vi "novoGoleiroAlinharComATrave.vi"(8 "balls":T1[](array[typedef]), 9 "Robot in":T2, 10 "Goleiro.X_padrao":dbl, 11 "IA State":T7={"our_robots"=[], "enemy_robots"=[], "balls"=[], "geometry"={"field_length"=0, "field_width"=0, "goal_width"=0, "goal_depth"=0, "center_circle_radius"=0, "defense_width"=0, "defense_depth"=0, "free_kick_from_defense_dist"=0, "penalty_spot_from_field_line_dist"=0, "penalty_line_from_spot_dist"=0, "half_moon_depth"=0, "half_moon_width"=0}, "IA Judge"={"stage"="", "command"="", "our_goalie_id"=0.0, "enemy_goalie_id"=0.0, "command enum"=enum."Halt", "Time"=enum."Azul"}, "Received Timestamp"=timestamp(0 s since 1904-01-01), "Events"={"Touch"=FALSE, "id touch"=0.0, "Ball out of \nVision"=FALSE, "Ball inside \nGoalie area"=FALSE, "Robot not responding"=FALSE, "Robots responding status"=[1.0, 1.0, 1.0, 1.0, 1.0, 1.0], "Enemy Ball \nPossession"=FALSE, "Id ini Possession"=0.0, "Ball Possesion"=FALSE, "Id Possesion"=0.0, "Ball at\nour goal side"=FALSE, "Ball at\ntouchline"=FALSE, "Ball at\nenemy goal side"=FALSE}}) -> (3 "Cluster de saída":T2)   [LabVIEW 2018]
uses:
  Core/AI Input.ctl
  Core/AI Robot.ctl
  Intel/Functions Enum.ctl
  Intel/AttackerStates.ctl
  Path Planning/RRT/PathDests.ctl
  Path Planning/RRT/PathDest.ctl
  Core/AI Ball.ctl
  Core/Field Size.ctl
  Core/AI Judge.ctl
  Intel/Command Enum.ctl
  Util/Events/Events.ctl
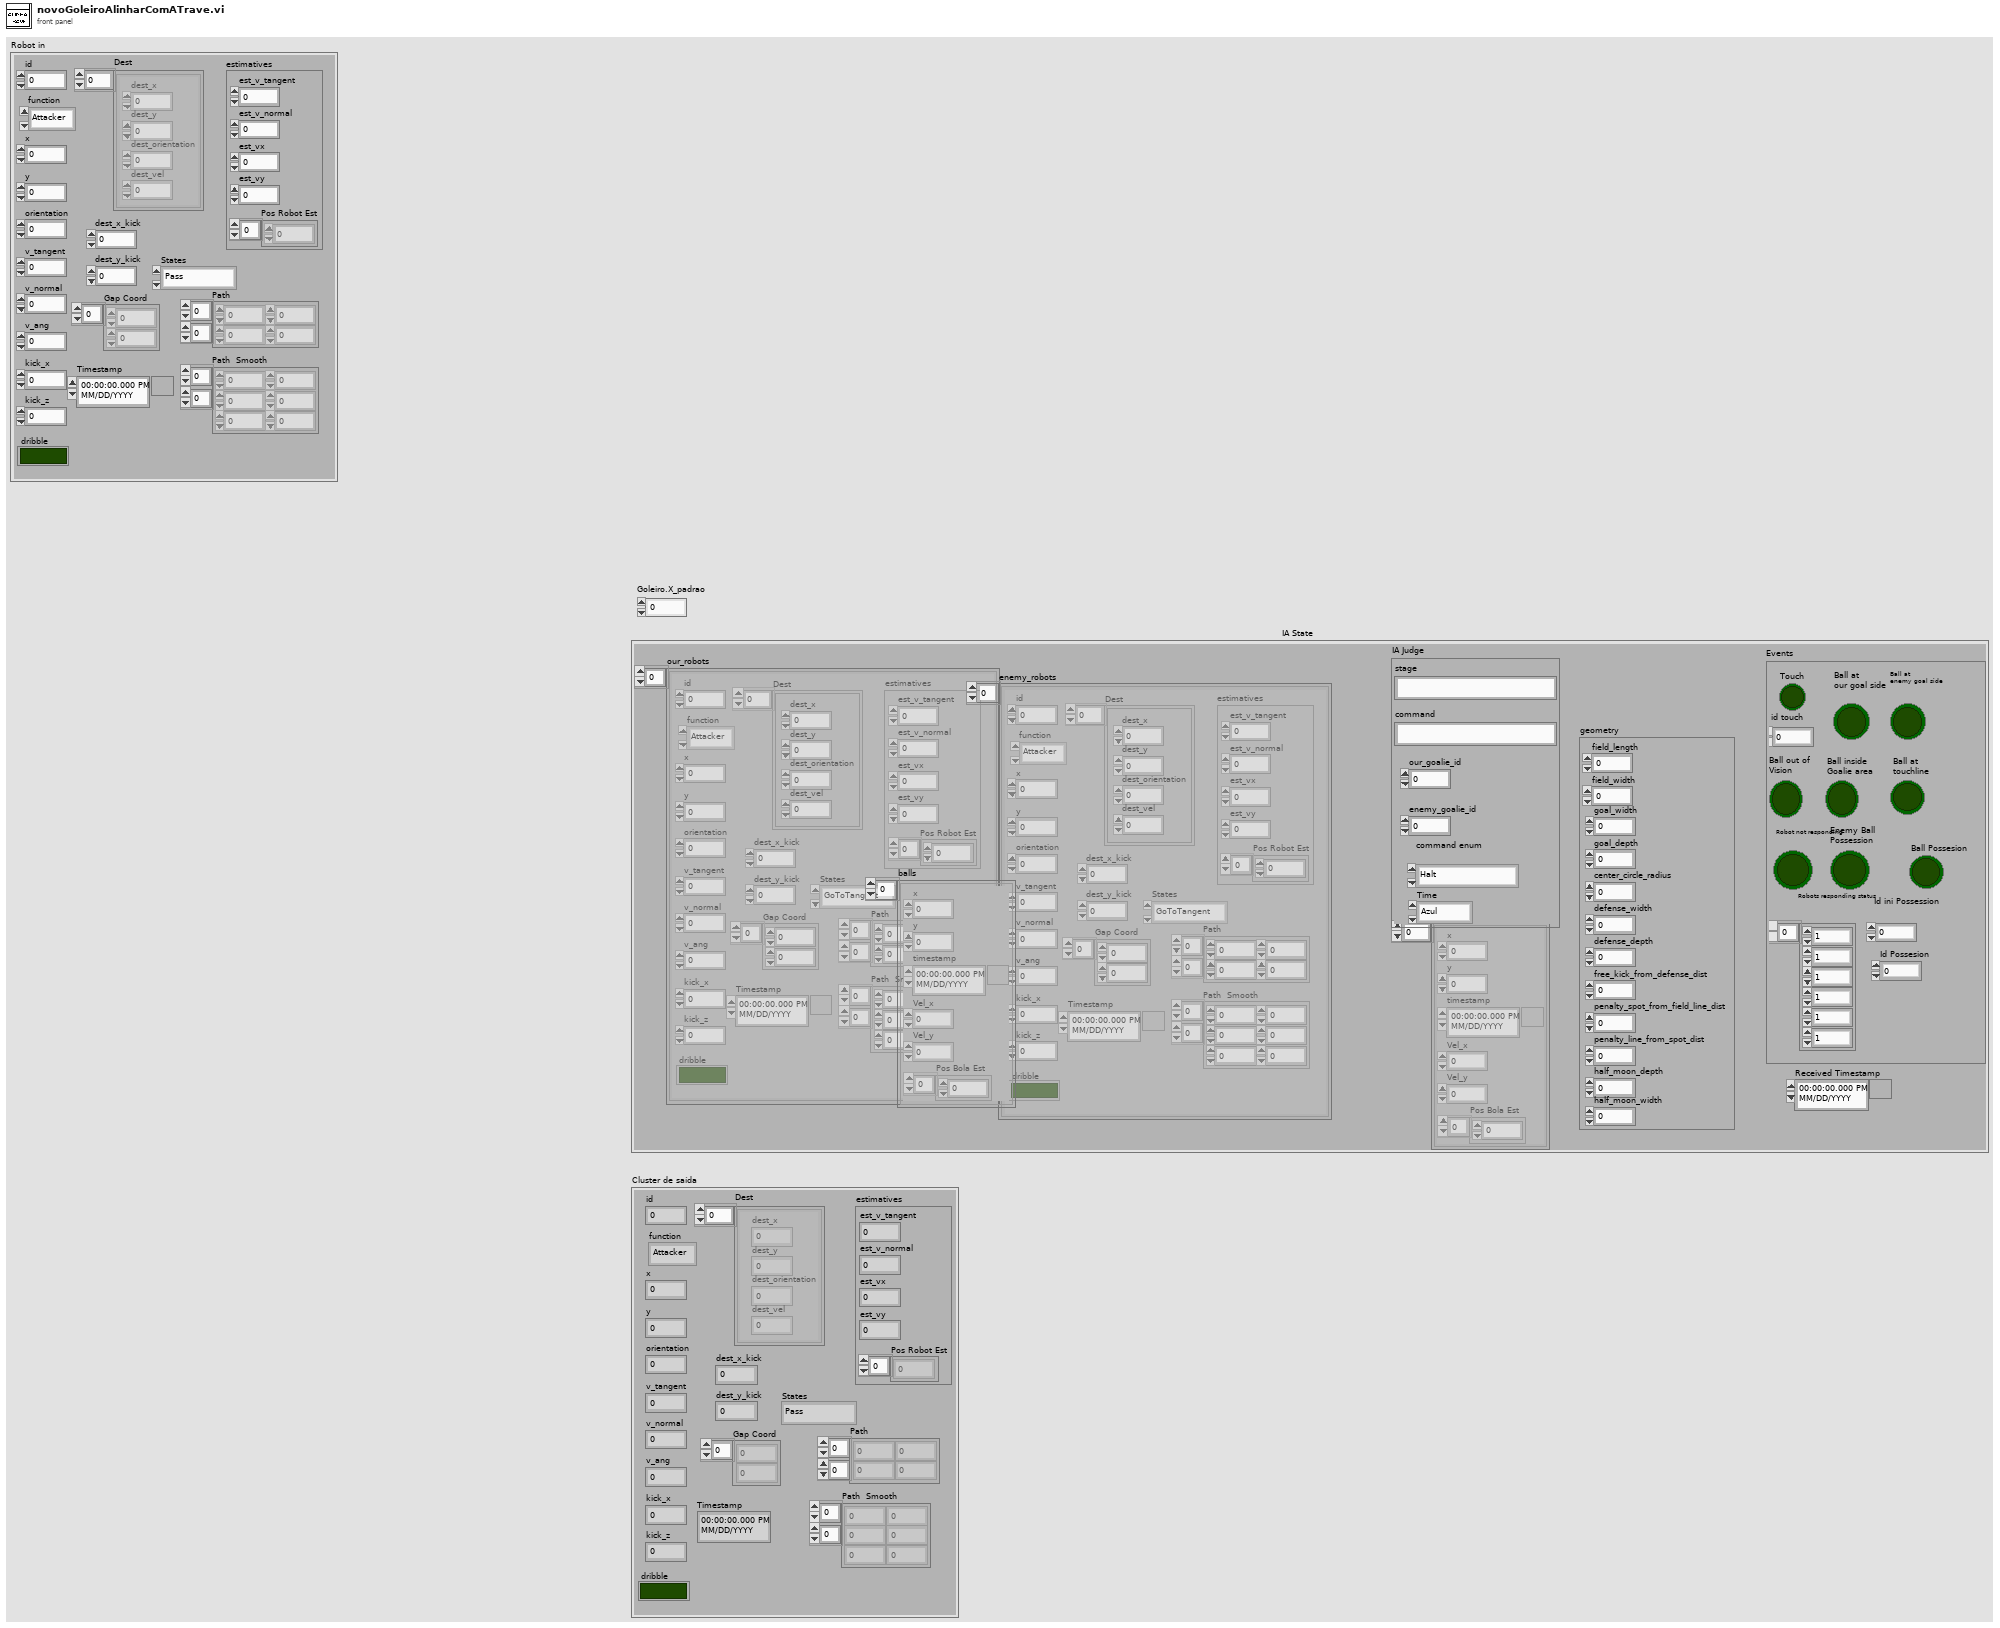
[diagram p1: front panel]
types:
  T1 = typedef "AI Ball.ctl" = cluster{"x":dbl, "y":dbl, "timestamp":timestamp, "Vel_x":dbl, "Vel_y":dbl, "Pos Bola Est":dbl[]}
  T2 = typedef "AI Robot.ctl" = cluster{"id":u32, "function":T3, "x":dbl, "y":dbl, "orientation":dbl, "v_tangent":dbl, "v_normal":dbl, "v_ang":dbl, "kick_x":dbl, "kick_z":dbl, "dribble":bool, "Timestamp":timestamp, "estimatives":cluster{"est_v_tangent":dbl, "est_v_normal":dbl, "est_vx":dbl, "est_vy":dbl, "Pos Robot Est":dbl[]}, "dest_x_kick":dbl, "dest_y_kick":dbl, "Gap Coord":dbl[], "States":T4, "Path ":dbl[][], "Path  Smooth":dbl[][], "Dest":T5}
  T3 = typedef "Functions Enum.ctl" = enum16{"Attacker", "Goalie", "Defender", "Striker", "Goto 0", "Dummy", "Kicker", "ZigZag"}
  T4 = typedef "AttackerStates.ctl" = enum16{"Pass", "GoToTangent", "BallGetting", "GoToKick", "Rotate anti-clockwise", "Rotate Clockwise", ""}
  T5 = typedef "PathDests.ctl" = T6[]
  T6 = typedef "PathDest.ctl" = cluster{"dest_x":dbl, "dest_y":dbl, "dest_orientation":dbl, "dest_vel":dbl}
  T7 = typedef "AI Input.ctl" = cluster{"our_robots":T2[], "enemy_robots":T2[], "balls":T1[], "geometry":T8, "IA Judge":T9, "Received Timestamp":timestamp, "Events":T11}
  T8 = typedef "Field Size.ctl" = cluster{"field_length":u32, "field_width":u32, "goal_width":u32, "goal_depth":u32, "center_circle_radius":u32, "defense_width":u32, "defense_depth":u32, "free_kick_from_defense_dist":u32, "penalty_spot_from_field_line_dist":u32, "penalty_line_from_spot_dist":u32, "half_moon_depth":u32, "half_moon_width":u32}
  T9 = typedef "AI Judge.ctl" = cluster{"stage":string, "command":string, "our_goalie_id":dbl, "enemy_goalie_id":dbl, "command enum":T10, "Time":enum16{"Azul", "Amarelo"}}
  T10 = typedef "Command Enum.ctl" = enum16{"Halt", "Stop", "Force Start", "PKA Normal Start", "Prepare Kickoff Ally", "PKE Normal Start", "Prepare Kickoff Enemy", "Prepare Penalty Ally", "PPA Normal Start", "Prepare Penalty Enemy", "PPE Normal Start", "Ball Placement Enemy Up", "Ball Placement Enemy Down", "Ball Placement Ally Up", "Ball Placement Ally Mid", "Ball Placement Ally Down", "Indirect Free Enemy", "Indirect Free Ally", "Timeout Enemy", "Timeout Ally", "Goal Enemy", "Goal Ally", "Normal Half Time", "Extra Time Break", "Extra Half Time", "None", "Post Game"}
  T11 = typedef "Events.ctl" = cluster{"Touch":bool, "id touch":dbl, "Ball out of \nVision":bool, "Ball inside \nGoalie area":bool, "Robot not responding":bool, "Robots responding status":dbl[], "Enemy Ball \nPossession":bool, "Id ini Possession":dbl, "Ball Possesion":bool, "Id Possesion":dbl, "Ball at\nour goal side":bool, "Ball at\ntouchline":bool, "Ball at\nenemy goal side":bool}
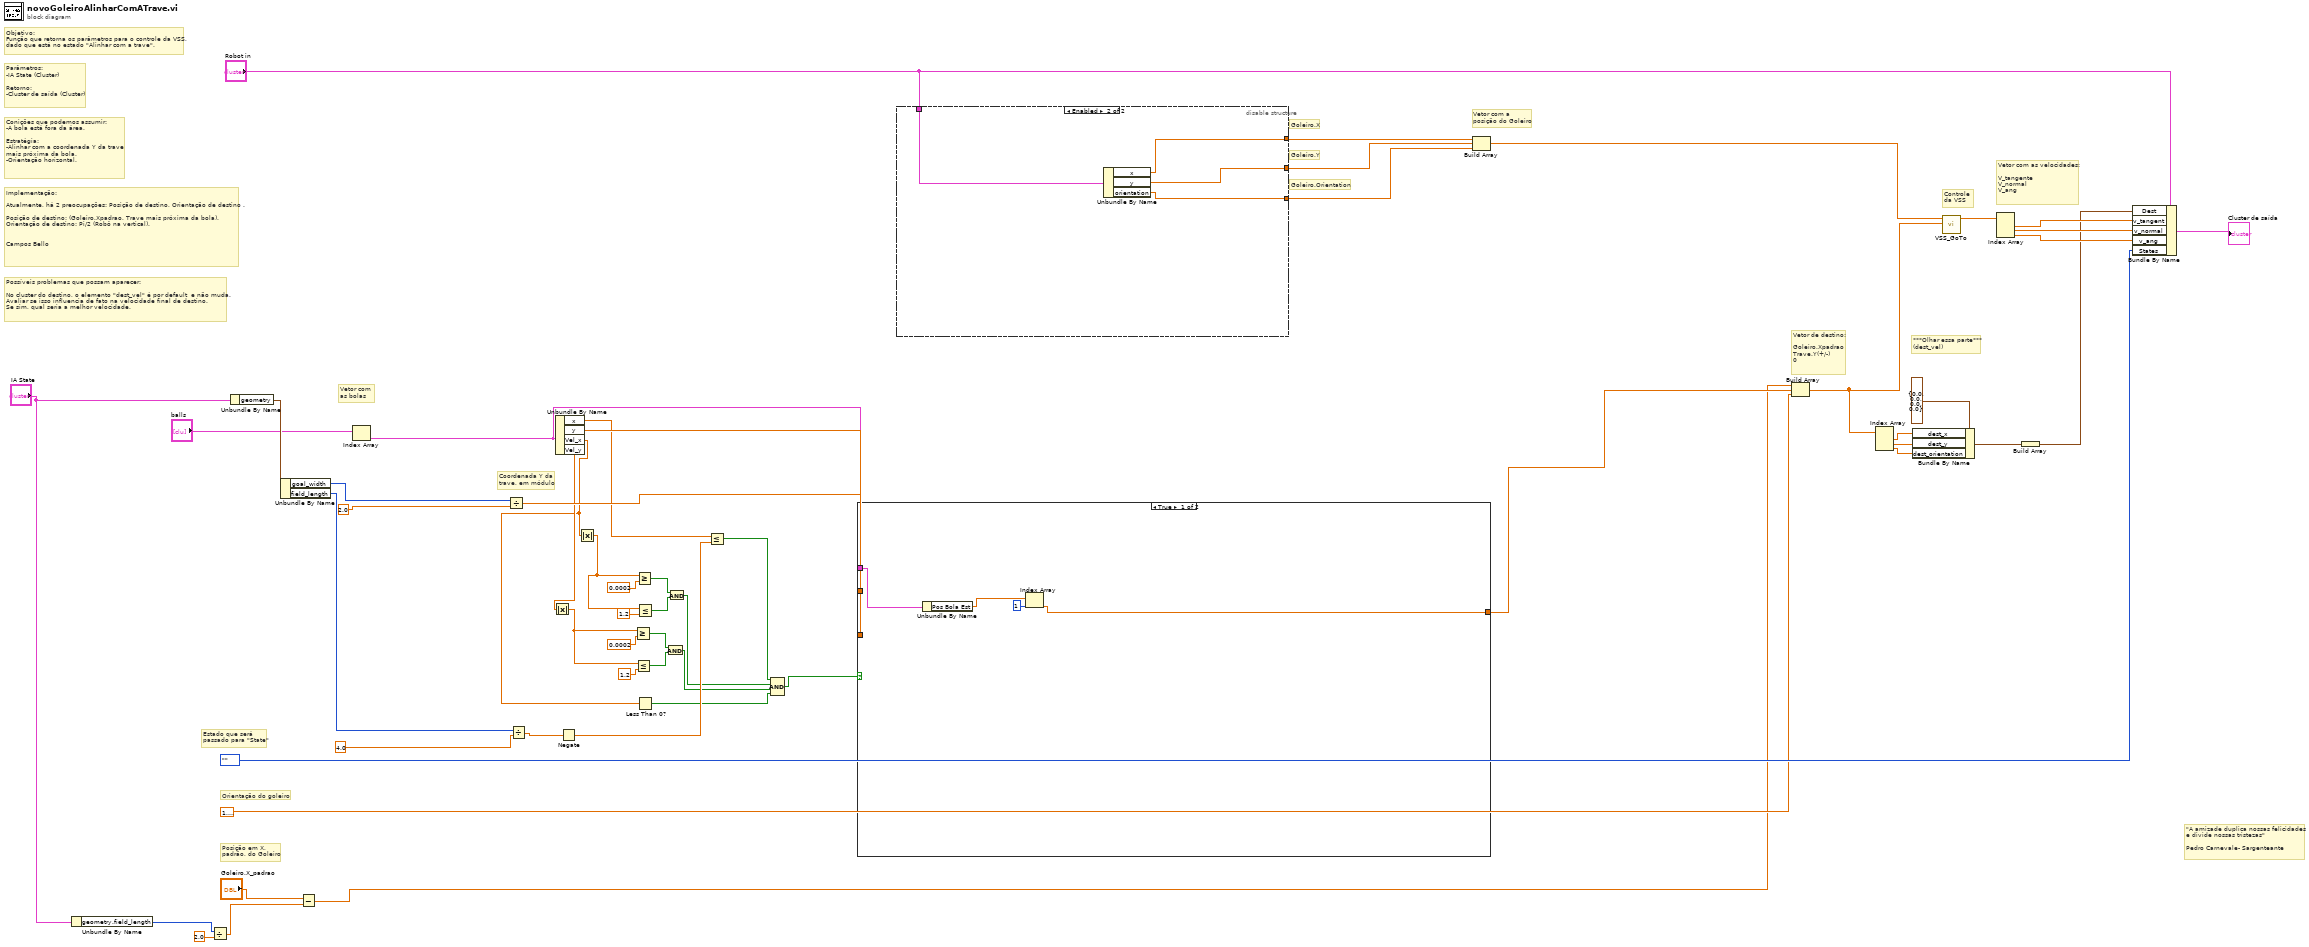
[diagram p0: block diagram]
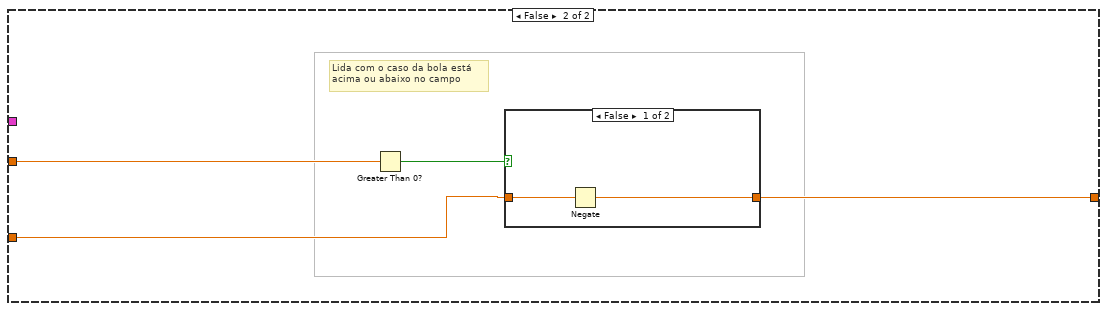
[diagram p2: hidden frame]
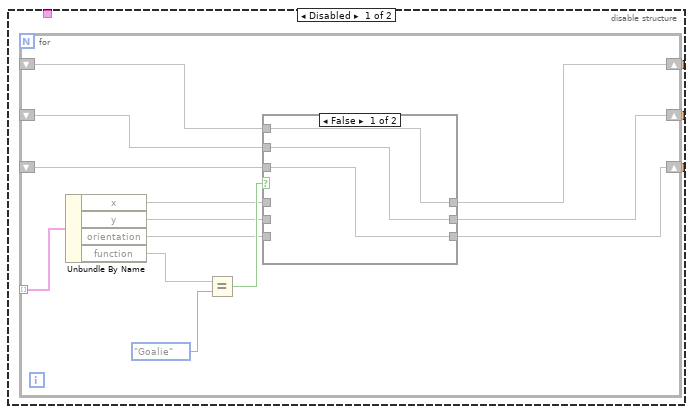
[diagram p4: hidden frame]
diagram:
  # "Coordenada Y da\ntrave, em módulo"
  # "\"A amizade duplica nossas felicidades \ne divide nossas tristezas\" \n\nPedro Carnevale- Sargenteante"
  # "Conições que podemos assumir:\n-A bola está fora da área.\n\nEstratégia:\n-Alinhar com a coordenada Y da trave \nmais próxima da bola.\n-Orientação horizontal."
  # "Possíveis problemas que possam aparecer:\n\nNo cluster do destino, o elemento \"dest_vel\" é por default  e não muda. \nAvaliar se isso influencia de fato na velocidade final de destino.\nSe sim, qual seria a melhor velocidade."
  # "Implementação:\n\nAtualmente, há 2 preocupações: Posição de destino, Orientação de destino .\n\nPosição de destino: (Goleiro.Xpadrao, Trave mais próxima da bola).\nOrientação de destino: Pi/2 (Robô na vertical).\n\n\nCampos Bello"
  # "Parâmetros:\n-IA State (Cluster)\n\nRetorno:\n-Cluster de saída (Cluster)"
  # "Objetivo:\nFunção que retorna os parâmetros para o controle da VSS,\ndado que está no estado \"Alinhar com a trave\"."
  # "Posição em X, \npadrão, do Goleiro"
  # "Orientação do goleiro"
  # "Estado que será\npassado para \"State\""
  # "Controle \nda VSS"
  # "***Olhar essa parte***\n(dest_vel)"
  # "Vetor com as velocidades:\n\nV_tangente\nV_normal\nV_ang"
  # "Vetor de destino:\n\nGoleiro.Xpadrao\nTrave.Y(+/-)\n0"
  # "Vetor com \nas bolas"
  # "Vetor com a \nposição do Goleiro"
  # "Goleiro.Orientation"
  # "Goleiro.Y"
  # "Goleiro.X"
  n1 = Unbundle By Name("IA State") -> ("geometry.field_length"=w28:u32)
  n2 = Divide(x=w28, y=2.0) -> (x/y=w27:dbl)
  n3 = Unbundle By Name("IA State") -> ("geometry"=w37:T8)
  n4 = Unbundle By Name(w37) -> ("goal_width"=w35:u32, "field_length"=w23:u32)
  n5 = Subtract(x="Goleiro.X_padrao", y=w27) -> (x-y=w26:dbl)
  n6 = Index Array(array="balls") -> (element=w20:T1)  [unwired: 1 in]
  n7 = Divide(x=w35, y=2.0 ("x/y")) -> (x/y=w34:dbl)
  n8 = Divide(x=w23, y=4.0) -> (x/y=w21:dbl)
  n9 = Unbundle By Name(w20) -> ("x"=w16:dbl, "y"=w38:dbl, "Vel_x"=w2:dbl, "Vel_y"=w7:dbl)
  n10 = Absolute Value(x=w7) -> (abs(x)=w6:dbl)
  n11 = Negate(x=w21) -> (-x=w17:dbl)
  n12 = Absolute Value(x=w2) -> (abs(x)=w8:dbl)
  n13 = Greater Or Equal?(x=w6, y=0.0002) -> (x >= y?=w12:bool)
  n14 = Less Or Equal?(x=w6, y=1.2) -> (x <= y?=w11:bool)
  n15 = Greater Or Equal?(x=w8, y=0.0002) -> (x >= y?=w15:bool)
  n16 = Less Or Equal?(x=w8, y=1.2) -> (x <= y?=w14:bool)
  n17 = Less Than 0?(x=w2) -> (x < 0?=w1:bool)
  n18 = And(x=w12, y=w11) -> (x .and. y?=w10:bool)
  n19 = And(x=w15, y=w14) -> (x .and. y?=w13:bool)
  n20 = Less Or Equal?(x=w16, y=w17) -> (x <= y?=w18:bool)
  n21 = Compound Arithmetic op=AND(w18, w13, w10, w1) -> (w19:bool)
  n22 = case shown="True" w19 {
    tunnel: w38 -> [_ w63]
    tunnel: w34 -> [_ w61]
    tunnel: [w56 w60] -> w33
    tunnel: w20 -> [w59 _]
    frame True {
      n23 = Unbundle By Name(w59) -> ("Pos Bola Est"=w58:dbl[])
      n24 = Index Array(array=w58, index=1) -> (element=w56:dbl)
    }
    frame False {
      # "Lida com o caso da bola está \nacima ou abaixo no campo"
      n25 = Greater Than 0?(x=w63) -> (x > 0?=w62:bool)
      n26 = case shown="False" w62 {
        tunnel: w61 -> [w65 w66]
        tunnel: [w64 w66] -> w60
        frame False {
          n27 = Negate(x=w65) -> (-x=w64:dbl)
        }
        frame True {
        }
      }
    }
  }
  n28 = disable-structure shown="Enabled" {
    disable-tunnel: [w70 w92] -> w55
    disable-tunnel: [w69 w90] -> w54
    disable-tunnel: [w68 w91] -> w53
    disable-tunnel: "Robot in" -> [_ w93]
    frame Disabled {
      n29 = for {
        tunnel: [w83] -> w67 mode=indexing
        shift-right: [w77] -> w70
        shift-left: _ -> [w75]
        shift-right: [w76] -> w68
        shift-left: _ -> [w74]
        shift-right: [w72] -> w69
        shift-left: _ -> [w71]
        n30 = Unbundle By Name(w83) -> ("x"=w79, "y"=w78, "orientation"=w73, "function"=w82)
        n31 = Equal?(x=w82, y=Functions_Enum."Goalie" ("function")) -> (x = y?=w80:bool)
        n32 = case shown="False" w80 {
          tunnel: w79 -> [_ w89]
          tunnel: w78 -> [_ w88]
          tunnel: [w86 w89] -> w77
          tunnel: [w85 w88] -> w76
          tunnel: w75 -> [w86 _]
          tunnel: w74 -> [w85 _]
          tunnel: w73 -> [_ w87]
          tunnel: [w84 w87] -> w72
          tunnel: w71 -> [w84 _]
          frame False {
          }
          frame True {
          }
        }
      }
    }
    frame Enabled {
      n33 = Unbundle By Name(w93) -> ("x"=w92:dbl, "y"=w91:dbl, "orientation"=w90:dbl)
    }
  }
  n34 = Build Array(w55, w53, w54) -> (w52:dbl[])
  n35 = Build Array(w26, w33, 1.5707963267948966) -> (w46:dbl[])
  n36 = Index Array(array=w46) -> (element #1=w45:dbl, element #2=w44:dbl, element #3=w43:dbl)  [unwired: 3 in]
  n37 = Bundle By Name(cluster=T6 {"dest_x"=0.0, "dest_y"=0.0, "dest_orientation"=0.0, "dest_vel"=0.0} ("element"), "dest_x"=w45, "dest_y"=w44, "dest_orientation"=w43) -> (w42:T6)
  n38 = call "VSS_GoTo.vi"("SetPoint"=w46, "Position"=w52) -> ("Output Vel"=w51:dbl[])  [unwired: 9 in]
  n39 = Index Array(array=w51) -> (element #1=w50:dbl, element #2=w49:dbl, element #3=w48:dbl)  [unwired: 3 in]
  n40 = Build Array(w42) -> (w41:T6[])
  n41 = Bundle By Name(cluster="Robot in", "Dest"=w41, "v_tangent"=w50, "v_normal"=w49, "v_ang"=w48, "States"=AttackerStates."") -> (→"Cluster de saída":T2)
